vi "Apply.vi"(8 "error in":errorcluster, 11 "DAQmx Base Configure Strategy in":refnum<class "DAQmx Base Configure Strategy.lvclass">) -> (0 "error out":errorcluster, 3 "DAQmx Base Configure Strategy out":refnum<class "DAQmx Base Configure Strategy.lvclass">)   [LabVIEW 2024, in "DAQmx Base Configure Strategy.lvclass"]
uses:
  DAQmx Base Configure Strategy.lvclass
  DAQmx Base Configure Strategy.lvclass/DAQmx Base Configure Strategy.ctl
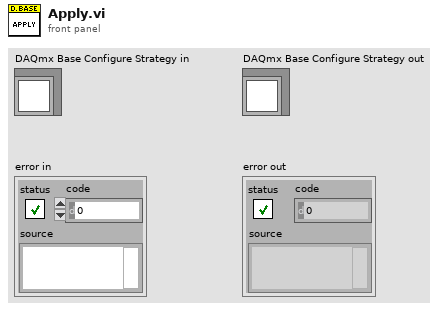
[diagram p1: front panel]
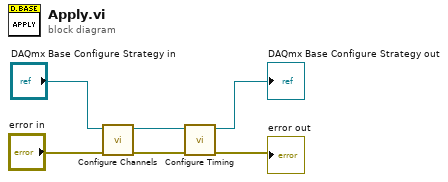
[diagram p0: block diagram]
diagram:
  n1 = call-dynamic "Configure Channels.vi"("error in"="error in", "DAQmx Base Configure Strategy in"="DAQmx Base Configure Strategy in") -> ("error out"=w5:errorcluster, "DAQmx Base Configure Strategy out"=w2:refnum<class "DAQmx Base Configure Strategy.lvclass">)  [unwired: 8 in]
  n2 = call-dynamic "Configure Timing.vi"("error in"=w5, "DAQmx Base Configure Strategy in"=w2) -> ("error out"=→"error out":errorcluster, "DAQmx Base Configure Strategy out"=→"DAQmx Base Configure Strategy out":refnum<class "DAQmx Base Configure Strategy.lvclass">)  [unwired: 8 in]
